vi "DefaultFromIni.vi"(8 "error in (no error)":errorcluster, 11 "PmuBase in":refnum<class "PmuBase.lvclass">) -> (0 "error out":errorcluster, 3 "PmuBase out":refnum<class "PmuBase.lvclass">)   [LabVIEW 2014, in "SensorPlugins.lvlib" / "PmuBase.lvclass"]
uses:
  PmuBase.lvclass
  Typedef/ePhases.ctl
  Typedef/PmuConfig.ctl
  <userlib>/NIST/BaseClasses/BasePlugin_class/BasePlugin.lvclass/BasePlugin.ctl
  PmuBase.lvclass/PmuBase.ctl
  Accessors/Write PhaseArray.vi
  Accessors/Write PmuConfig.vi
  <userlib>/NIST/BaseClasses/BasePlugin_class/Accessors/Read PluginIniFilePath.vi
  <vilib>/Utility/error.llb/Error Cluster From Error Code.vi
  <vilib>/ErrorRing/Error Ring.xnode
  <vilib>/Utility/config.llb/NI_LVConfig.lvlib
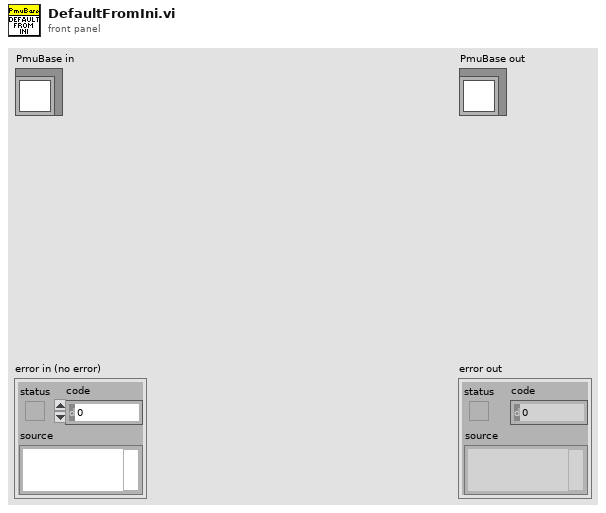
[diagram p1: front panel]
types:
  T1 = typedef "SensorPlugins.lvlib/PmuBase.lvclass/PmuConfig.ctl" = cluster{"Class":enum16{"M", "P"}, "Fs":i32, "F0":i32, "FSamp":i32, "SettlingTime":dbl, "T0":ext}
  T2 = typedef "SensorPlugins.lvlib/PmuBase.lvclass/ePhases.ctl" = enum16{"VA", "VB", "VC", "V+", "IA", "IB", "IC", "I+", "none"}
  T3 = typedef "NI_LVConfig.lvlib/Config Data RefNum.ctl" = refnum<k1>
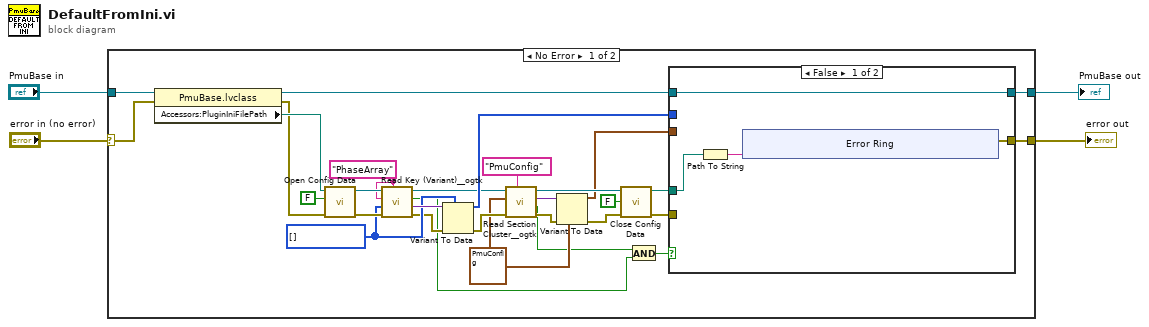
[diagram p0: block diagram]
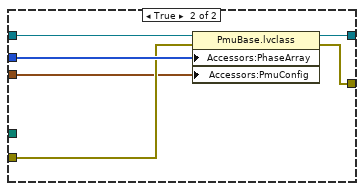
[diagram p2: hidden frame]
diagram:
  n1 = case shown="No Error" "error in (no error)" {
    selector: "error in (no error)" -> [w33 w52]
    tunnel: "PmuBase in" -> [w34 w53]
    tunnel: [w26 w53] -> w2
    tunnel: [w21 w52] -> w1
    frame No Error {
      w11 = T1 {"Class"=enum."M", "Fs"=60, "F0"=60, "FSamp"=60, "SettlingTime"=0.0, "T0"=0.0} ("PmuConfig")
      w18 = "PhaseArray" ("section")
      w24 = T2[] [] items=["VA", "VB", "VC", "V+", "IA", "IB", "IC", "I+", "none"]
      n2 = property class="PmuBase.lvclass"(reference=w34, error in=w33) -> (reference out=w27:refnum<class "PmuBase.lvclass">, error out=w30:errorcluster, "Accessors:PluginIniFilePath"=w32:path)
      n3 = call <vilib>:"Open Config Data.vi"("error in (no error)"=w30, "create file if necessary (T)"=FALSE, "configuration file path"=w32) -> ("error out"=w28:errorcluster, "refnum"=w29:T3)  [unwired: 6 in, 1 out]
      n4 = call <userlib>:"Read Key (Variant)__ogtk.vi"("section"=w18, "error in (no error)"=w28, "type"=w24, "key (optional)"=w18, "refnum"=w29) -> ("error out"=w23:errorcluster, "key-value"=w25:variant, "found?"=w6:bool, "refnum out"=w17:T3)  [unwired: 3 in]
      n5 = Variant To Data(error in=w23, type=w24, Variant=w25) -> (data=w22:T2[], error out=w15:errorcluster)
      n6 = call <userlib>:"Read Section Cluster__ogtk.vi"("section (optional)"="PmuConfig", "error in (no error)"=w15, "Section Formatted Cluster Type"=w11, "refnum"=w17) -> ("error out"=w13:errorcluster, "all found?"=w7:bool, "Section Formatted Cluster"=w12:variant, "dup refnum"=w16:T3)  [unwired: 3 in, 1 out]
      n7 = Variant To Data(error in=w13, type=w11, Variant=w12) -> (data=w9:T1, error out=w10:errorcluster)
      n8 = call <vilib>:"Close Config Data.vi"("error in (no error)"=w10, "write file if changed (T)"=FALSE, "refnum"=w16) -> ("error out"=w20:errorcluster, "file path"=w5:path)  [unwired: 7 in]
      n9 = And(x=w7, y=w6) -> (x .and. y?=w8:bool)
      n10 = case shown="False" w8 {
        tunnel: w27 -> [w38 w51]
        tunnel: [w38 w50] -> w26
        tunnel: w22 -> [_ w49]
        tunnel: [w35 w48] -> w21
        tunnel: w20 -> [_ w47]
        tunnel: w9 -> [_ w46]
        tunnel: w5 -> [w36 _]
        frame False {
          n11 = Path To String(path=w36) -> (string=w37:string)
          n12 = xnode "Error Ring"("parameter 0"=w37) -> ("error out"=w35:errorcluster)
        }
        frame True {
          n13 = property class="PmuBase.lvclass"(reference=w51, error in=w47, "Accessors:PhaseArray"=w49, "Accessors:PmuConfig"=w46) -> (reference out=w50:refnum<class "PmuBase.lvclass">, error out=w48:errorcluster)
        }
      }
    }
    frame Error {
    }
  }
  "error out" <- w1
  "PmuBase out" <- w2
